vi "RTD Range.vi"() -> ()   [LabVIEW 2020, in "Yokogawa GX Series.lvlib"]
uses:
  <instrlib>/Yokogawa GX Series/Yokogawa GX Series.lvlib
panel:
  in  "RTD Range":string="Pt100\nPt100-H\nJPt100\nJPt100-H\nCu10GE\nCu10LN\nCu10WEED\nCu10BAILEY\nCu10a392\nCu10a393\nCu25\nCu53\nCu100\nJ263B\nNi100SAMA\nNi100DIN\nNi120\nPt25\nPt50\nPt200WEED\nCu10G\nCu50G\nCu100G\nPt46G\nPt100G"
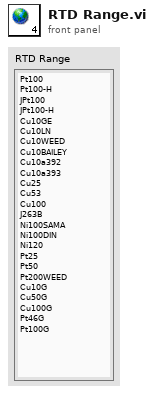
[diagram p1: front panel]
diagram:
